vi "Msg.vi"(7 "jettl in":refnum<class "jettl.lvclass">, 11 "Setup Msg Strategy in":refnum<class "Setup Msg Strategy.lvclass">) -> (5 "jettl out":refnum<class "jettl.lvclass">)   [LabVIEW 2021, in "jettl.lvlib" / "Setup Msg Strategy.lvlib" / "Setup Msg Strategy.lvclass"]
uses:
  Setup Msg Strategy.lvclass
  Setup Msg Strategy.lvclass/Setup Msg Strategy.ctl
  Setup/Setup.lvclass
  jettl/jettl.lvclass
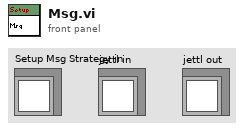
[diagram p1: front panel]
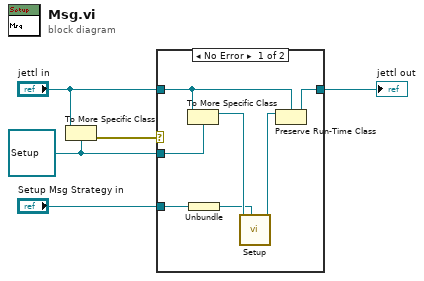
[diagram p0: block diagram]
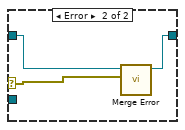
[diagram p2: hidden frame]
diagram:
  w3 = refnum<class "Setup.lvclass"> refnum ("Setup.lvlib:Setup.lvclass")
  n1 = To More Specific Class(target class=w3, reference="jettl in") -> (error out=w5:errorcluster)  [unwired: 1 in, 1 out]
  n2 = case shown="No Error" w5 {
    selector: w5 -> [_ w14]
    tunnel: [w10 w13] -> w2
    tunnel: "jettl in" -> [w11 w15]
    tunnel: w3 -> [w12 _]
    tunnel: "Setup Msg Strategy in" -> [w7 _]
    frame No Error {
      n3 = To More Specific Class(target class=w12, reference=w11) -> (specific class reference=w9:refnum<class "Setup.lvclass">)  [unwired: 1 in, 1 out]
      n4 = Unbundle "Unbundle"(w7) -> (w6:refnum<class "Sender.lvclass">)
      n5 = call-dynamic "Setup.vi"("Sender"=w6, "Setup in"=w9) -> ("Setup out"=w8:refnum<class "Setup.lvclass">)  [unwired: 9 in]
      n6 = Preserve Run-Time Class(object in=w8, 2:w11) -> (object out=w10:refnum<class "jettl.lvclass">)  [unwired: 1 in, 1 out]
    }
    frame Error {
      n7 = call-dynamic "Merge Error.vi"("Error"=w14, "jettl in"=w15) -> ("jettl out"=w13:refnum<class "jettl.lvclass">)  [unwired: 9 in]
    }
  }
  "jettl out" <- w2
